vi "Write Message Stream.vi"(10 "Message Stream":refnum<class "Message Stream.lvclass">, 11 "Network Endpoint in":refnum<class "Network Endpoint.lvclass">) -> (3 "Network Endpoint out":refnum<class "Network Endpoint.lvclass">)   [LabVIEW 2020, in "Network Endpoint.lvlib" / "Network Endpoint.lvclass"]
doc: "Use this accessor to specify the Message Stream that will be used for the connection. You must set this value prior to launching the actor."
uses:
  Network Endpoint.lvclass
  Abstract Classes/Message Stream/Message Stream.lvclass
  Network Endpoint.lvclass/Network Endpoint.ctl
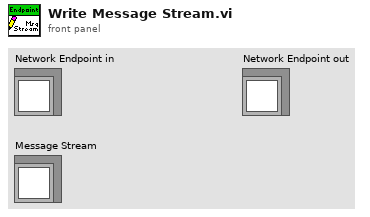
[diagram p1: front panel]
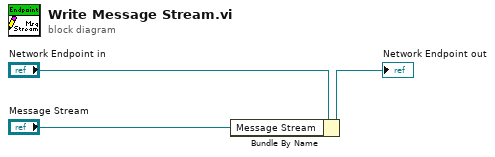
[diagram p0: block diagram]
diagram:
  n1 = Bundle By Name(cluster="Network Endpoint in", "Message Stream"="Message Stream") -> (→"Network Endpoint out":refnum<class "Network Endpoint.lvclass">)
